vi "Serial Transmit.vi"(6 "transfer length":u8, 7 "serial clock shift edge (falling)":enum16{"rising", "falling"}(ring)=enum."falling", 8 "transmit":bool, 9 "input valid":bool, 10 "serial clock in":bool, 11 "sample":u32) -> (3 "data bit out":bool, 4 "ready for input":bool)   [LabVIEW 2013, in "I2S-TDM.lvlib"]
uses:
  I2S-TDM.lvlib
  Controls/serial transmit states.ctl
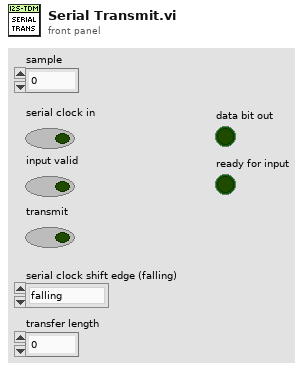
[diagram p1: front panel]
types:
  T1 = typedef "I2S-TDM.lvlib/serial transmit states.ctl" = enum16{"idle", "transfer"}
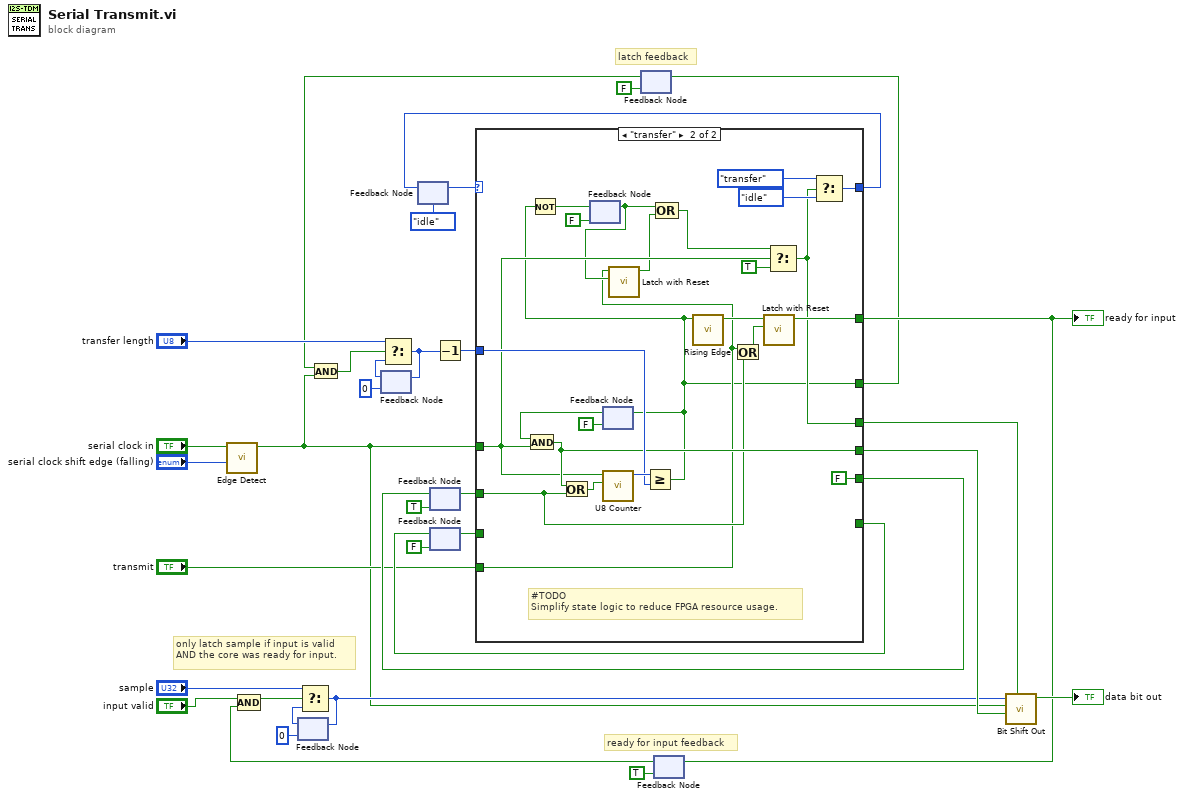
[diagram p0: block diagram]
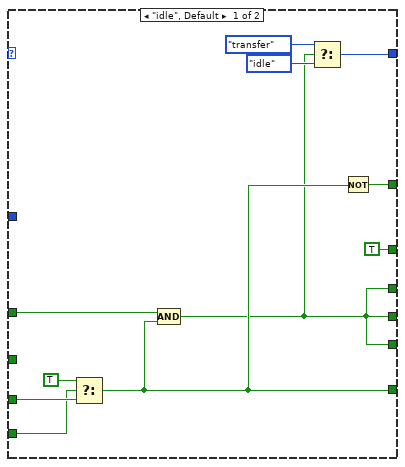
[diagram p2: hidden frame]
diagram:
  # "latch feedback"
  # "ready for input feedback"
  # "only latch sample if input is valid AND the core was ready for input."
  n1 = call "Edge Detect.vi"("edge (rising)"="serial clock shift edge (falling)", "signal in"="serial clock in") -> ("edge detected?"=w4:bool)  [unwired: 9 in]
  n2 = feedback #1(u32 0 ("sample")) -> (w17:u32)
  n3 = feedback #2(u8 0 ("sample")) -> (w13:u8)
  n4 = feedback #3(serial_transmit_states."idle" ("transmit state")) -> (w33:T1)
  n5 = feedback #4(TRUE ("transmit")) -> (w28:bool)
  n6 = feedback #5(FALSE ("transmit")) -> (w26:bool)
  n7 = feedback #6(FALSE) -> (w3:bool)
  n8 = And(x=w3, y=w4) -> (x .and. y?=w1:bool)
  n9 = Select(t="transfer length", s=w1, f=w13) -> (s? t:f=w11:u8)
  n10 = feedback-in #2(w11) -> ()
  n11 = Decrement(x=w11) -> (x-1=w23:u8)
  n12 = case shown="\"transfer\"" w33 {
    tunnel: [w45 w66] -> w19
    tunnel: w4 -> [w43 w57]
    tunnel: w23 -> [_ w64]
    tunnel: [w36 w50] -> w30
    tunnel: w28 -> [_ w49]
    tunnel: [w36 FALSE] -> w22
    tunnel: "transmit" -> [w39 w48]
    tunnel: w26 -> [w41 _]
    tunnel: [w38 _] -> w25
    tunnel: [w37 w58] -> w10
    tunnel: [w36 w60] -> w21
    tunnel: [TRUE w46] -> w5
    frame "idle", Default {
      n13 = Select(t=TRUE, s=w39, f=w41) -> (s? t:f=w38:bool)
      n14 = Compound Arithmetic op=AND(w43, w38) -> (w36:bool)
      n15 = Select(t=serial_transmit_states."transfer", s=w36, f=serial_transmit_states."idle" ("transmit state")) -> (s? t:f=w45:T1)
      n16 = Not(x=w38) -> (.not. x?=w37:bool)
    }
    frame "transfer" {
      # "#TODO\nSimplify state logic to reduce FPGA resource usage."
      n17 = feedback #7(FALSE) -> (w52:bool)
      n18 = feedback #8(FALSE) -> (w63:bool)
      n19 = And(x=w63, y=w57) -> (x .and. y?=w60:bool)
      n20 = Or(x=w60, y=w49) -> (x .or. y?=w61:bool)
      n21 = call "U8 Counter.vi"("reset (F)"=w61, "increment"=w57) -> ("count"=w69:u8)  [unwired: 9 in]
      n22 = call "Latch with Reset.vi"("reset"=w52, "signal"=w48) -> ("latched signal"=w51:bool)  [unwired: 9 in]
      n23 = Greater Or Equal?(x=w69, y=w64) -> (x >= y?=w46:bool)
      n24 = Not(x=w46) -> (.not. x?=w55:bool)
      n25 = feedback-in #7(w55) -> ()
      n26 = feedback-in #8(w46) -> ()
      n27 = Compound Arithmetic op=OR(w52, w51) -> (w53:bool)
      n28 = call "Rising Edge.vi"("signal in"=w46) -> ("rising edge?"=w65:bool)  [unwired: 10 in]
      n29 = Or(x=w48, y=w49) -> (x .or. y?=w47:bool)
      n30 = call "Latch with Reset.vi"("reset"=w47, "signal"=w65) -> ("latched signal"=w58:bool)  [unwired: 9 in]
      n31 = Select(t=w53, s=w57, f=TRUE) -> (s? t:f=w50:bool)
      n32 = Select(t=serial_transmit_states."transfer" ("transmit state"), s=w50, f=serial_transmit_states."idle" ("transmit state")) -> (s? t:f=w66:T1)
    }
  }
  "ready for input" <- w10
  n33 = feedback-in #3(w19) -> ()
  n34 = feedback-in #4(w22) -> ()
  n35 = feedback-in #5(w25) -> ()
  n36 = feedback-in #6(w5) -> ()
  n37 = feedback-in #9(w10) -> ()
  n38 = feedback #9(TRUE ("latched signal")) -> (w8:bool)
  n39 = Compound Arithmetic op=AND("input valid", w8) -> (w6:bool)
  n40 = Select(t="sample", s=w6, f=w17) -> (s? t:f=w18:u32)
  n41 = feedback-in #1(w18) -> ()
  n42 = call "Bit Shift Out.vi"("output enable"=w30, "reset"=w21, "shift bits"=w4, "sample"=w18) -> ("bit out"=→"data bit out":bool)  [unwired: 7 in]
